vi "Signals (Set).vi"   [LabVIEW 2013, in "Mercury iXX.lvlib"]
doc: "Set the signal data of any devices within the Mercury Instrument."
uses:
  <instrlib>/Mercury iXX/Mercury iXX.lvlib
  <instrlib>/Mercury iXX/Public/Libraries/Heater.lvlib
  <instrlib>/Mercury iXX/Public/Libraries/Magnet.lvlib
  <instrlib>/Mercury iXX/Public/Libraries/Auxiliary.lvlib
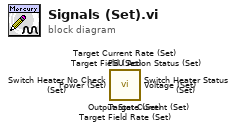
[diagram p0: block diagram]
diagram:
  n1 = call <instrlib>:"Output State (Set).vi"() -> ()  [unwired: 8 in, 4 out]
  n2 = call <instrlib>:"PSU Action Status (Set).vi"() -> ()  [unwired: 8 in, 4 out]
  n3 = call <instrlib>:"Switch Heater No Check (Set).vi"() -> ()  [unwired: 8 in, 4 out]
  n4 = call <instrlib>:"Switch Heater Status (Set).vi"() -> ()  [unwired: 8 in, 4 out]
  n5 = call <instrlib>:"Target Field Rate (Set).vi"() -> ()  [unwired: 8 in, 4 out]
  n6 = call <instrlib>:"Target Current Rate (Set).vi"() -> ()  [unwired: 8 in, 4 out]
  n7 = call <instrlib>:"Target Field (Set).vi"() -> ()  [unwired: 8 in, 4 out]
  n8 = call <instrlib>:"Target Current (Set).vi"() -> ()  [unwired: 8 in, 4 out]
  n9 = call <instrlib>:"Power (Set).vi"() -> ()  [unwired: 8 in, 4 out]
  n10 = call <instrlib>:"Voltage (Set).vi"() -> ()  [unwired: 8 in, 4 out]
